vi "Encender_led_cam.vi"(8 "error in (no error)":errorcluster) -> (0 "error out":errorcluster, 3 "reference out":refnum<k7>)   [LabVIEW 2019]
panel:
  in  "DNVideoX":refnum<k7>(container)
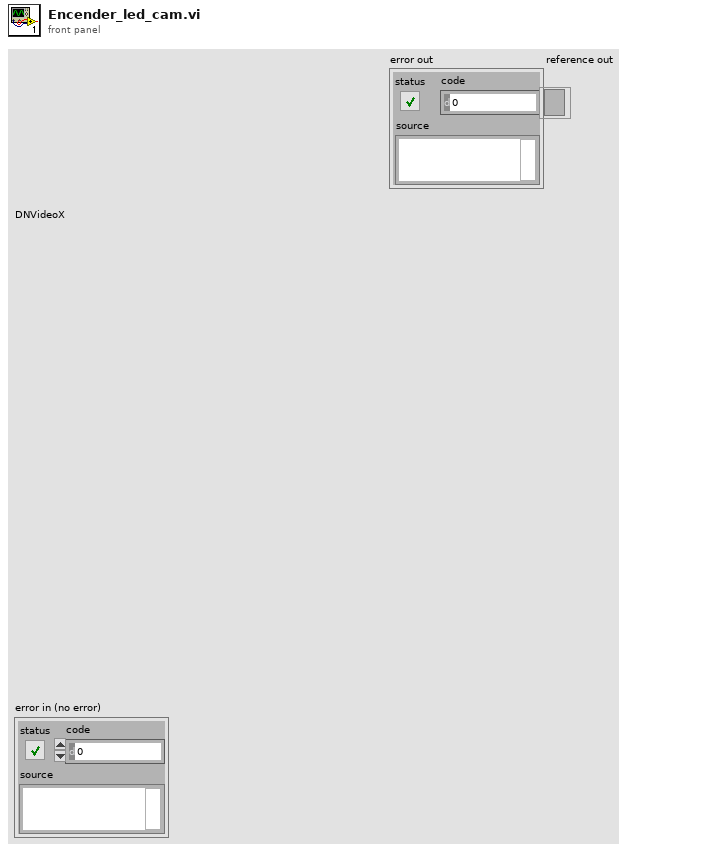
[diagram p1: front panel]
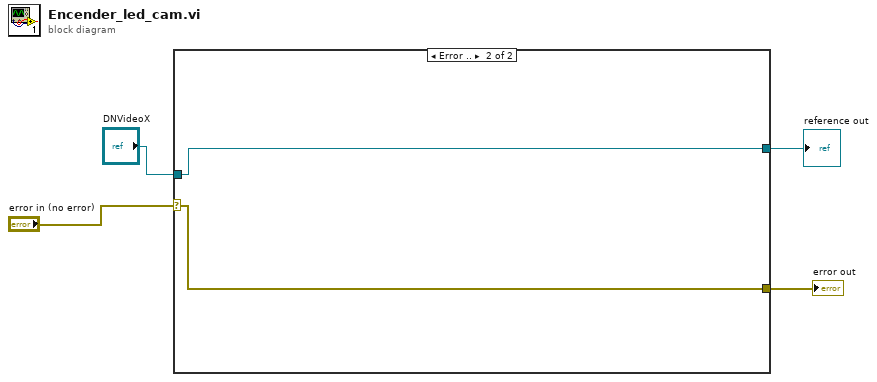
[diagram p0: block diagram]
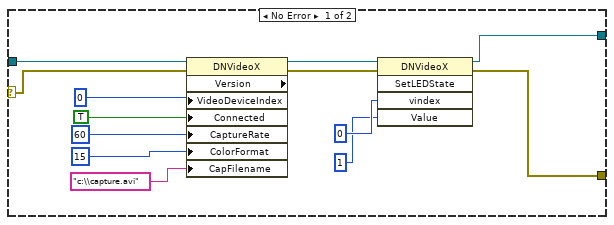
[diagram p2: hidden frame]
diagram:
  n1 = case shown="Error .." "error in (no error)" {
    selector: "error in (no error)" -> [w5 w19]
    tunnel: [w8 w19] -> w4
    tunnel: [w7 w18] -> w3
    tunnel: "DNVideoX" -> [w6 w18]
    frame No Error {
      n2 = property class="DNVideoX" props=["Version", "VideoDeviceIndex", "Connected", "CaptureRate", "ColorFormat", "CapFilename"](reference=w6, error in=w5, "VideoDeviceIndex"=0, "Connected"=TRUE, "CaptureRate"=60 ("VideoDeviceIndex"), "ColorFormat"=15 ("VideoDeviceIndex"), "CapFilename"="c:\\capture.avi" ("default name")) -> (reference out=w10:refnum<k7>, error out=w9:errorcluster)  [unwired: 1 out]
      n3 = invoke class="DNVideoX" method="SetLEDState"(reference=w10, error in=w9, "vindex"=0, "Value"=1) -> (reference out=w7:refnum<k7>, error out=w8:errorcluster)  [unwired: 1 in, 3 out]
    }
    frame Error {
    }
  }
  "error out" <- w4
  "reference out" <- w3
